vi "all.vi"() -> ()   [LabVIEW 2012]
uses:
  SubVIs/typedef/User Accounts.ctl
  SubVIs/typedef/Log_User_Data.ctl
  SubVIs/typedef/User_Data_Cluster.ctl
panel:
  out "Array out":string[](array[string])
  in  "Account":T1
  in  "Log Cluster":T2
  in  "User-data cluster":T3
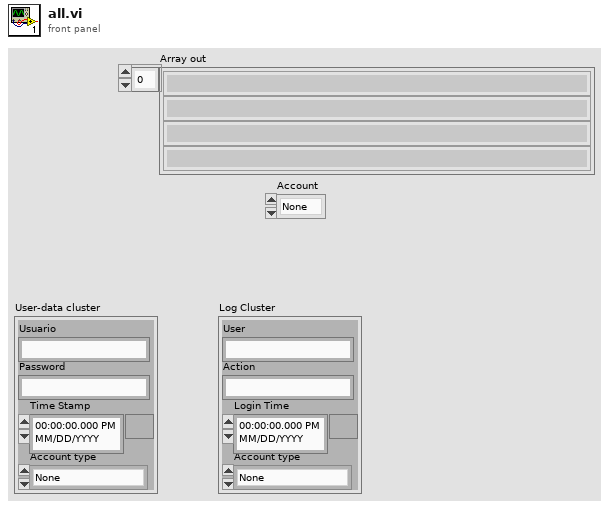
[diagram p1: front panel]
types:
  T1 = typedef "User Accounts.ctl" = enum16{"None", "User", "Admin"}
  T2 = typedef "Log_User_Data.ctl" = cluster{"User":string, "Action":string, "Account type":T1, "Login Time ":timestamp}
  T3 = typedef "User_Data_Cluster.ctl" = cluster{"Usuario":string, "Password":string, "Account type":T1, "Time Stamp":timestamp}
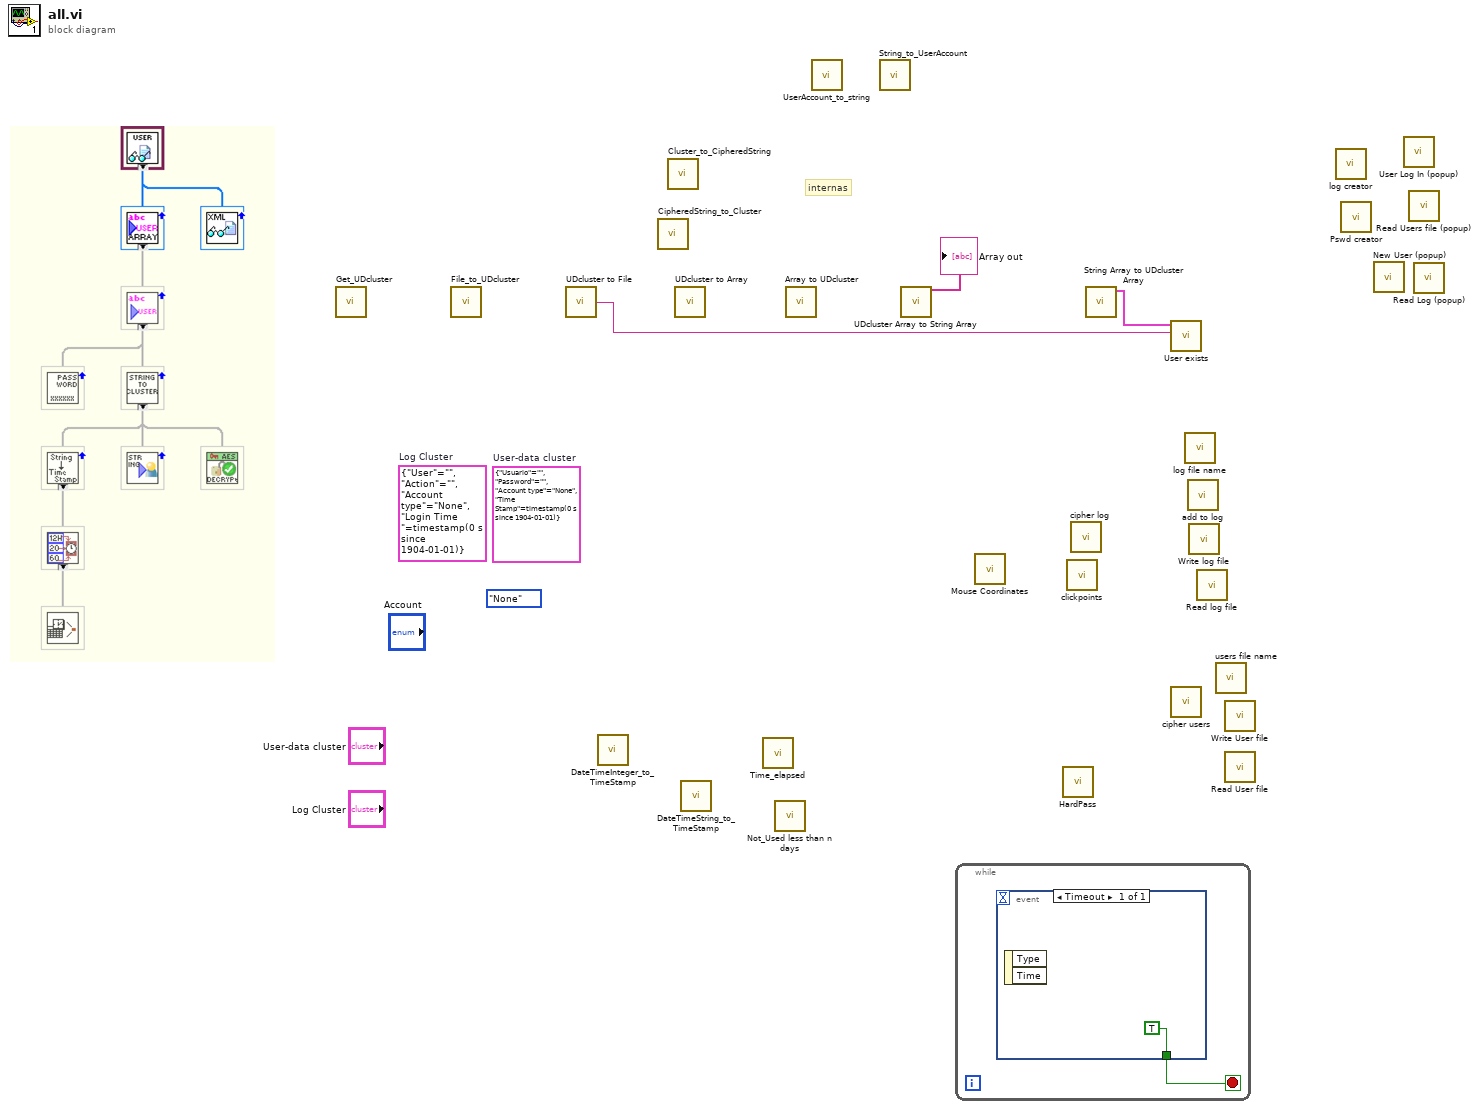
[diagram p0: block diagram]
diagram:
  (unwired) User_Accounts."None" ("Account")
  (unwired) T3 {"Usuario"="", "Password"="", "Account type"=enum."None", "Time Stamp"=timestamp(0 s since 1904-01-01)}  # User-data cluster
  (unwired) T2 {"User"="", "Action"="", "Account type"=enum."None", "Login Time "=timestamp(0 s since 1904-01-01)}  # Log Cluster
  # "internas"
  n1 = call "Get_UDcluster.vi"() -> ()  [unwired: 14 in, 2 out]
  n2 = call "File_to_UDcluster.vi"() -> ()  [unwired: 14 in, 2 out]
  n3 = call "UDcluster to File.vi"() -> ("CypheredText"=w2:string)  [unwired: 1 in]
  n4 = call "DateTimeInteger_to_TimeStamp.vi"() -> ()  [unwired: 19 in, 1 out]
  n5 = call "CipheredString_to_Cluster.vi"() -> ()  [unwired: 11 in, 5 out]
  n6 = call "Cluster_to_CipheredString.vi"() -> ()  [unwired: 14 in, 2 out]
  n7 = call "UDcluster to Array.vi"() -> ()  [unwired: 14 in, 2 out]
  n8 = call "DateTimeString_to_TimeStamp.vi"() -> ()  [unwired: 10 in, 2 out]
  n9 = call "Time_elapsed.vi"() -> ()  [unwired: 8 in, 4 out]
  n10 = call "Not_Used less than n days.vi"() -> ()  [unwired: 10 in, 2 out]
  n11 = call "Array to UDcluster.vi"() -> ()  [unwired: 14 in, 2 out]
  n12 = call "UserAccount_to_string.vi"() -> ()  [unwired: 1 in, 1 out]
  n13 = call "String_to_UserAccount.vi"() -> ()  [unwired: 1 in, 1 out]
  n14 = call "UDcluster Array to String Array.vi"() -> ("Array out"=→"Array out":string[])  [unwired: 14 in, 1 out]
  n15 = while {
    stop <- w4 stop-if-true
    n16 = event shown="[0] Timeout" {
      selector: _ -> [_]
      dyn-events: _ -> [_]
      timeout: _ -> [_]
      tunnel: [TRUE] -> w4
      event Timeout {
        n17 = event-data() -> ()  [unwired: 1 in, 2 out]
      }
    }
  }
  n18 = call "Mouse Coordinates.vi"() -> ()  [unwired: 1 in]
  n19 = call "HardPass.vi"() -> ()  [unwired: 12 in, 4 out]
  n20 = call "clickpoints.vi"() -> ()  [unwired: 9 in, 3 out]
  n21 = call "cipher log.vi"() -> ()  [unwired: 15 in, 1 out]
  n22 = call "String Array to UDcluster Array.vi"() -> ("Array"=w3:T3[])  [unwired: 10 in, 1 out]
  n23 = call "User exists.vi"("user"=w2, "Array"=w3) -> ()  [unwired: 6 in, 4 out]
  n24 = call "cipher users.vi"() -> ()  [unwired: 11 in, 1 out]
  n25 = call "log file name.vi"() -> ()  [unwired: 15 in, 1 out]
  n26 = call "add to log.vi"() -> ()  [unwired: 16 in]
  n27 = call "Write log file.vi"() -> ()  [unwired: 10 in, 2 out]
  n28 = call "Read log file.vi"() -> ()  [unwired: 14 in, 2 out]
  n29 = call "users file name.vi"() -> ()  [unwired: 15 in, 1 out]
  n30 = call "Write User file.vi"() -> ()  [unwired: 10 in, 2 out]
  n31 = call "Read User file.vi"() -> ()  [unwired: 14 in, 2 out]
  n32 = call "log creator.vi"() -> ()  [unwired: 12 in]
  n33 = call "Pswd creator.vi"() -> ()  [unwired: 12 in]
  n34 = call "New User (popup).vi"() -> ()  [unwired: 11 in, 1 out]
  n35 = call "User Log In (popup).vi"() -> ()  [unwired: 10 in, 2 out]
  n36 = call "Read Users file (popup).vi"() -> ()  [unwired: 15 in, 1 out]
  n37 = call "Read Log (popup).vi"() -> ()  [unwired: 11 in, 1 out]
